vi "Corr_stats_labels.vi"(2 "Inst 2 Units":T1={"Colour"=0, "Inst type"=enum."Pitot-static tube", "Inst name"="Manometer voltage", "Symbol"="U", "Code name"="", "Extra Info"="U", "Inst Array"=enum."PWA", "U"=0.0, "u^2"=0.0, "u^3"=0.0, "u^4"=0.0, "Skew_u"=0.0, "Kurt_u"=0.0, "Sd Error in Mean"=0.0, "% u'/U"=0.0, "X"=0.0, "Y"=0.0, "Z"=0.0, "Timescale integral Estimate"=0.0, "Sd Error in Variance"=0.0, "Calib File"=path "", "Calib Constants"=[], "Output Position"=FALSE, "Stats"=enum."None", "Av Sampling Rate"=0.0, "Av No of Samples"=0.0, "Total Meas Time (s)"=0.0, "OrigChName"="", "Max value"=0.0, "Min value"=0.0, "Req Sample Rate Hz"=0.0, "Sync Delay Time (s)"=0.0, "Ch No"=0, "Device"="", "Use Latest Calib"=FALSE, "Port"="", "Metadata Ch Names"=[], "Metadata Ch Values"=[], "Label"="", "chState"=enum."Solo", "Point Drift"=0.0, "inputConfig"=""} {"Kurt_u" format="%_3g"; "u^4" format="%_3g"; "u^3" format="%_3g"; "Sd Error in Variance" format="%_3g"; "u^2" format="%_3g"; "Sd Error in Mean" format="%_3g"; "U" format="%_3g"; "Sync Delay Time (s)" format="%.4f"; "Total Meas Time (s)" format="%_5g"; "Skew_u" format="%_3g"; "% u'/U" format="%_3g"}, 3 "Inst 1 Units":T1={"Colour"=0, "Inst type"=enum."Pitot-static tube", "Inst name"="Manometer voltage", "Symbol"="U", "Code name"="", "Extra Info"="U", "Inst Array"=enum."PWA", "U"=0.0, "u^2"=0.0, "u^3"=0.0, "u^4"=0.0, "Skew_u"=0.0, "Kurt_u"=0.0, "Sd Error in Mean"=0.0, "% u'/U"=0.0, "X"=0.0, "Y"=0.0, "Z"=0.0, "Timescale integral Estimate"=0.0, "Sd Error in Variance"=0.0, "Calib File"=path "", "Calib Constants"=[], "Output Position"=FALSE, "Stats"=enum."None", "Av Sampling Rate"=0.0, "Av No of Samples"=0.0, "Total Meas Time (s)"=0.0, "OrigChName"="", "Max value"=0.0, "Min value"=0.0, "Req Sample Rate Hz"=0.0, "Sync Delay Time (s)"=0.0, "Ch No"=0, "Device"="", "Use Latest Calib"=FALSE, "Port"="", "Metadata Ch Names"=[], "Metadata Ch Values"=[], "Label"="", "chState"=enum."Solo", "Point Drift"=0.0, "inputConfig"=""} {"Kurt_u" format="%_3g"; "u^4" format="%_3g"; "u^3" format="%_3g"; "Sd Error in Variance" format="%_3g"; "u^2" format="%_3g"; "Sd Error in Mean" format="%_3g"; "U" format="%_3g"; "Sync Delay Time (s)" format="%.4f"; "Total Meas Time (s)" format="%_5g"; "Skew_u" format="%_3g"; "% u'/U" format="%_3g"}) -> (0 "Output":string[](array[string]))   [LabVIEW 2022 SP3]
uses:
  Globals/Meas_global.vi
  Controls/Inst_type.ctl
  Controls/Analysis_info_cluster.ctl
  Controls/Instrument_Array.ctl
  Controls/channelState.ctl
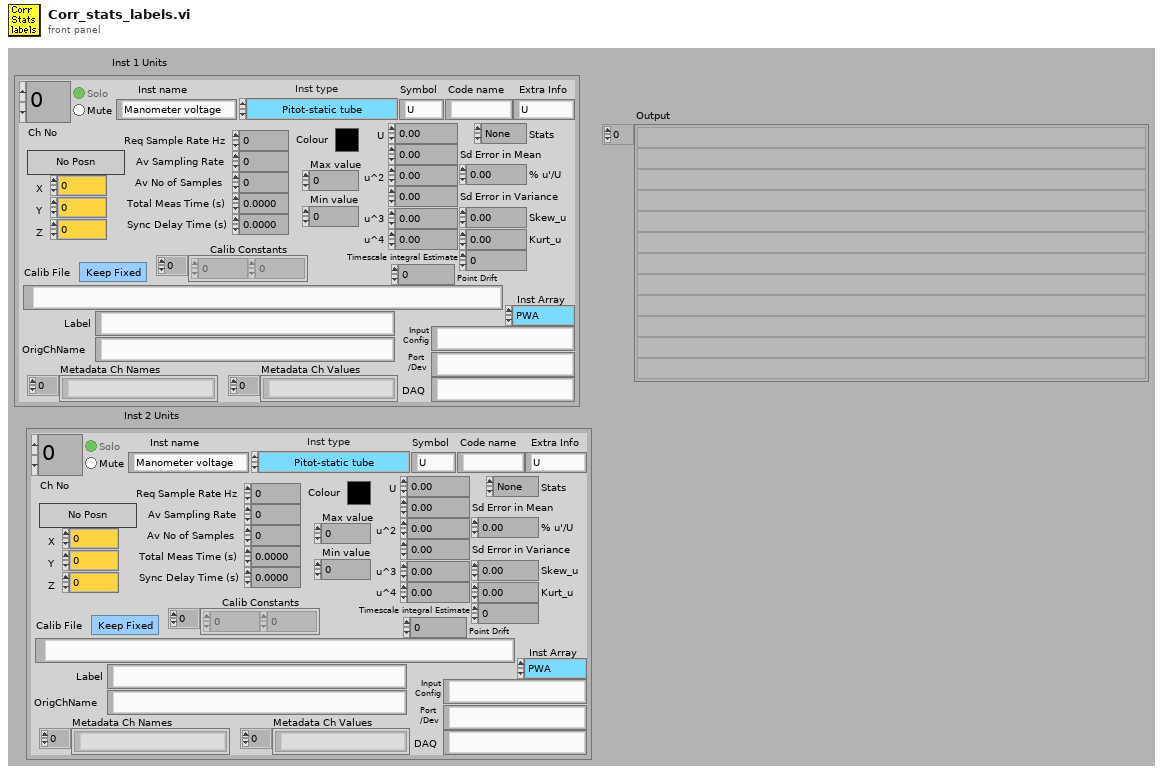
[diagram p1: front panel]
types:
  T1 = typedef "Analysis_info_cluster.ctl" = cluster{"Colour":u32, "Inst type":T2, "Inst name":string, "Symbol":string, "Code name":string, "Extra Info":string, "Inst Array":T3, "U":dbl, "u^2":dbl, "u^3":dbl, "u^4":dbl, "Skew_u":dbl, "Kurt_u":dbl, "Sd Error in Mean":dbl, "% u'/U":dbl, "X":dbl, "Y":dbl, "Z":dbl, "Timescale integral Estimate":dbl, "Sd Error in Variance":dbl, "Calib File":path, "Calib Constants":dbl[], "Output Position":bool, "Stats":enum16{"None", "Basic", "Full"}, "Av Sampling Rate":dbl, "Av No of Samples":dbl, "Total Meas Time (s)":dbl, "OrigChName":string, "Max value":dbl, "Min value":dbl, "Req Sample Rate Hz":dbl, "Sync Delay Time (s)":dbl, "Ch No":i16, "Device":string, "Use Latest Calib":bool, "Port":string, "Metadata Ch Names":string[], "Metadata Ch Values":string[], "Label":string, "chState":T4, "Point Drift":dbl, "inputConfig":string}
  T2 = typedef "Inst_type.ctl" = enum16{"Raw voltage", "Raw with zero offsetting", "Propeller anemometer", "Pressure Transducer", "Pitot-static tube", "Hot wire", "Cross wire 1", "Cross wire 2", "Generic Linear", "Generic Polynomial", "Generic BackPoly", "Fast FID", "Thermocouple", "Cold wire", "Pulsed Wire", "LDA Vel", "LDA Tran time", "LDA Arr time", "Microphone"}
  T3 = typedef "Instrument_Array.ctl" = enum16{"PWA", "LDA", "Analogue"}
  T4 = typedef "channelState.ctl" = enum32{"No Selection", "Solo", "Mute"}
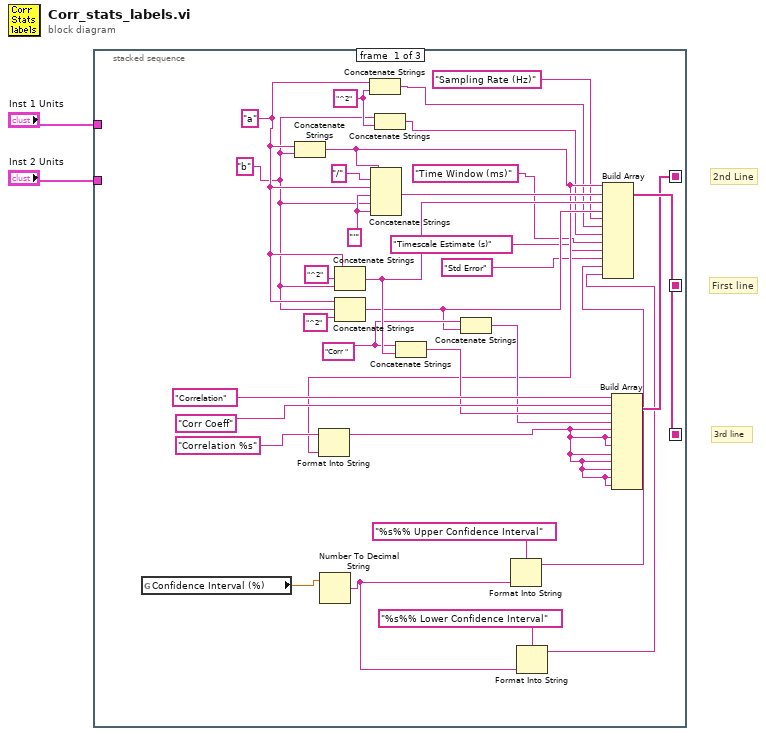
[diagram p0: block diagram]
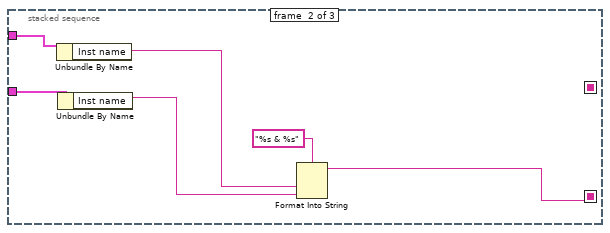
[diagram p2: hidden frame]
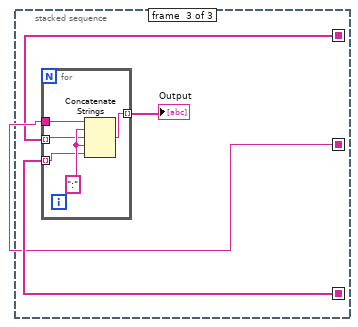
[diagram p3: hidden frame]
diagram:
  # "First line"
  # "2nd Line"
  # "3rd line"
  n1 = stacked-sequence {
    seq-local: [w32 _ _] -> [_ _ w44]
    seq-local: [w31 _ _] -> [_ _ w41]
    seq-local: [_ w35 _] -> [_ _ w42]
    tunnel: "Inst 2 Units" -> [_ w39 _]
    tunnel: "Inst 1 Units" -> [_ w40 _]
    frame #0 {
      w3 = "b"
      w4 = "a"
      w10 = "^2"
      w23 = "Corr "
      w27 = "'"
      n2 = global read "Meas_global.vi" "Confidence Interval (%)"() -> (w19:dbl)
      n3 = Concatenate Strings(w4, w3) -> (w17:string)
      n4 = Format Into String(format string="Correlation %s", w17) -> (resulting string=w7:string)  [unwired: 2 in, 1 out]
      n5 = Number To Decimal String(number=w19) -> (decimal integer string=w15:string)  [unwired: 1 in]
      n6 = Concatenate Strings(w4, "^2", w3) -> (w25:string)
      n7 = Concatenate Strings(w4, w3, "^2") -> (w22:string)
      n8 = Concatenate Strings(w4, w10) -> (w9:string)
      n9 = Concatenate Strings(w17, "/", w4, w27, w3, w27) -> (w26:string)
      n10 = Concatenate Strings(w3, w10) -> (w8:string)
      n11 = Concatenate Strings(w23, w25) -> (w24:string)
      n12 = Concatenate Strings(w23, w22) -> (w21:string)
      n13 = Format Into String(format string="%s%% Upper Confidence Interval", w15) -> (resulting string=w14:string)  [unwired: 2 in, 1 out]
      n14 = Format Into String(format string="%s%% Lower Confidence Interval", w15) -> (resulting string=w13:string)  [unwired: 2 in, 1 out]
      n15 = Build Array(w17, w26, w25, w22, "Sampling Rate (Hz)", w9, w8, "Time Window (ms)", "Timescale Estimate (s)", "Std Error", w14, w13) -> (w32:string[])
      n16 = Build Array("Correlation", "Corr Coeff", w24, w21, w7, w7, w7, w7, w7, w7, w7, w7) -> (w31:string[])
    }
    frame #1 {
      n17 = Unbundle By Name(w40) -> ("Inst name"=w37:string)
      n18 = Unbundle By Name(w39) -> ("Inst name"=w36:string)
      n19 = Format Into String(format string="%s & %s" ("Format String"), w37, w36) -> (resulting string=w35:string)  [unwired: 2 in, 1 out]
    }
    frame #2 {
      n20 = for {
        tunnel: [w49] -> w43 mode=indexing
        tunnel: w42 -> [w48]
        tunnel: w41 -> [w46] mode=indexing
        tunnel: w44 -> [w45] mode=indexing
        w47 = ":" ("Substring")
        n21 = Concatenate Strings(w48, w47, w46, w47, w45) -> (w49:string)
      }
      "Output" <- w43
    }
  }
